vi "Autonomous_Thread.vi"   [LabVIEW 2011]
doc: "This VI is called when autonomous begins, and will automatically be terminated when autonomous ends. You can carry out timed or sensor driven robot movement independently without needing to return to the caller."
uses:
  MutexMode.ctl
  Auto_Conf.vi
panel:
  # "Each item in this array is an autonomous script file.\nThis array is indexed by the autoMode variable in Robot Global Data."
types:
  T1 = typedef "MutexMode.ctl" = enum16{"Get Mode", "Request Execution", "Stop Execution", "Lock Autonomous", "Script Completed"}
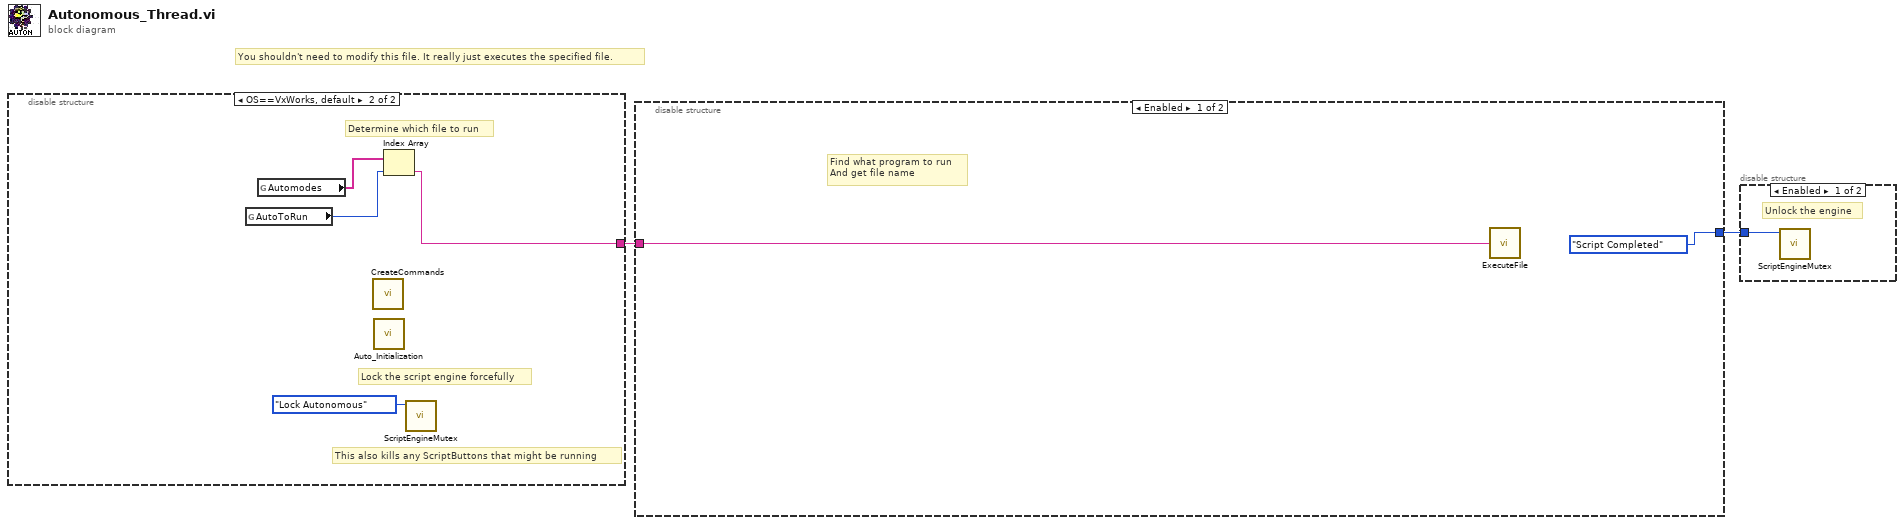
[diagram p0: block diagram]
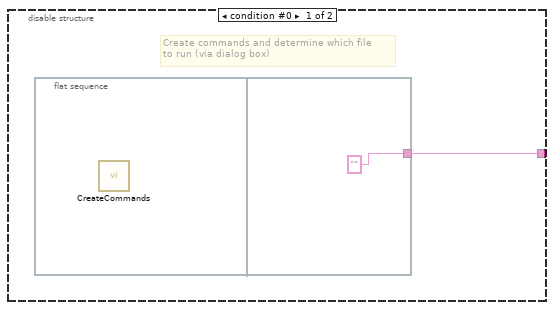
[diagram p3: hidden frame]
diagram:
  # "You shouldn't need to modify this file. It really just executes the specified file."
  n1 = disable-structure shown="OS==VxWorks, default" {
    disable-tunnel: [w3 w6] -> w2
    frame condition #0 {
      # "Create commands and determine which file\nto run (via dialog box)"
      n2 = flat-sequence {
        tunnel: ["" ("File Name With Extension")] -> w3
        frame #0 {
          n3 = call "CreateCommands.vi"() -> ()  [unwired: 1 out]
        }
        frame #1 {
        }
      }
    }
    frame condition #1 (active) {
      # "This also kills any ScriptButtons that might be running"
      # "Lock the script engine forcefully"
      # "Determine which file to run"
      n4 = global read "Auto_Conf.vi" "AutoToRun"() -> (w8:u8)
      n5 = global read "Auto_Conf.vi" "Automodes"() -> (w5:string[])
      n6 = call "CreateCommands.vi"() -> ()  [unwired: 1 out]
      n7 = call "Auto_Initialization.vi"() -> ()  [unwired: 1 out]
      n8 = Index Array(array=w5, index=w8) -> (element=w6:string)
      n9 = call "ScriptEngineMutex.vi"("Mutex Mode"=MutexMode."Lock Autonomous") -> ()  [unwired: 10 in, 1 out]
    }
  }
  n10 = disable-structure shown="Enabled" {
    disable-tunnel: w2 -> [w10 _]
    disable-tunnel: [MutexMode."Script Completed" ("Mutex Mode") _] -> w1
    frame Enabled {
      # "Find what program to run\nAnd get file name"
      n11 = call "ExecuteFile.vi"("File Name With Extension"=w10) -> ()
    }
    frame Disabled {
    }
  }
  n12 = disable-structure shown="Enabled" {
    disable-tunnel: w1 -> [w11 _]
    frame Enabled {
      # "Unlock the engine"
      n13 = call "ScriptEngineMutex.vi"("Mutex Mode"=w11) -> ()  [unwired: 10 in, 1 out]
    }
    frame Disabled {
    }
  }
